vi "NIDCPower_channel_ganging - check channel list_full config.vi"(8 "error in (no error)":errorcluster, 11 "Channel List In":T1[](array[typedef])) -> (0 "error out":errorcluster, 3 "Channel List Out":T1[](array[typedef]))   [LabVIEW 2024]
uses:
  ctl/NIDCPower_channel_ganging - ctl - channel def.ctl
  ctl/NIDCPower_channel_ganging - ctl - channel mode.ctl
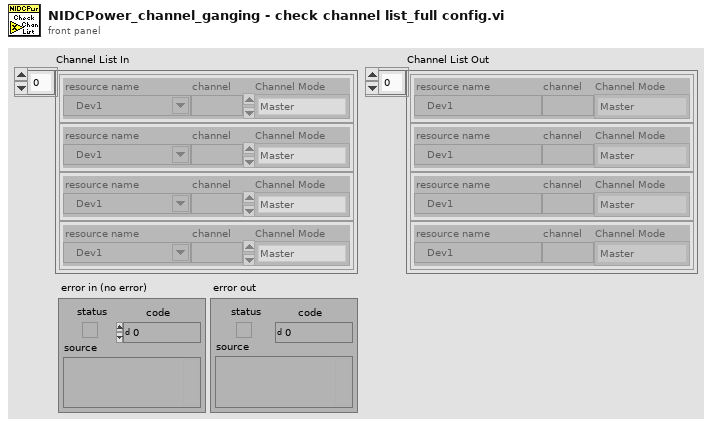
[diagram p1: front panel]
types:
  T1 = typedef "NIDCPower_channel_ganging - ctl - channel def.ctl" = cluster{"resource name":refnum<k15>, "channels":string, "Channel Mode":T2}
  T2 = typedef "NIDCPower_channel_ganging - ctl - channel mode.ctl" = enum32{"Master", "Slave", "Slave - Inverted"}
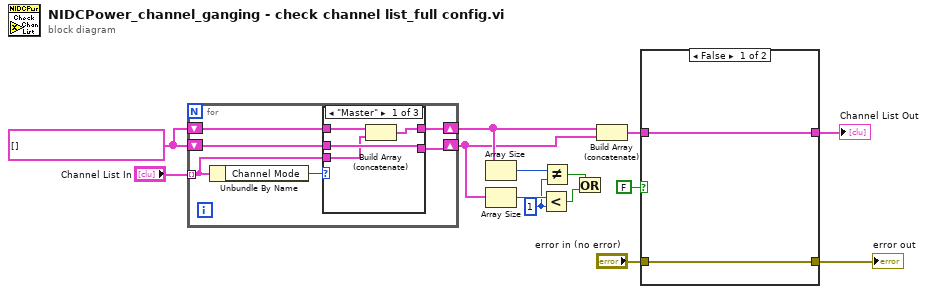
[diagram p0: block diagram]
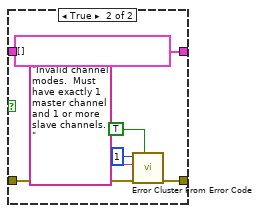
[diagram p2: hidden frame]
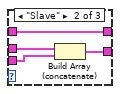
[diagram p3: hidden frame]
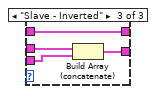
[diagram p4: hidden frame]
diagram:
  w10 = 1 ("y")
  w13 = T1[] [] ("Channel List")
  n1 = for {
    tunnel: "Channel List In" -> [w16] mode=indexing
    shift-right: [w15] -> w6
    shift-left: w13 -> [w17]
    shift-right: [w18] -> w7
    shift-left: w13 -> [w19]
    n2 = Unbundle By Name(w16) -> ("Channel Mode"=w20:T2)
    n3 = case shown="\"Master\"" w20 {
      tunnel: w19 -> [w23 w28 w32]
      tunnel: [w22 w28 w32] -> w18
      tunnel: w17 -> [w24 w27 w31]
      tunnel: w16 -> [w21 w26 w30]
      tunnel: [w24 w25 w29] -> w15
      frame "Master" {
        n4 = Build Array (concatenate)(w23, w21) -> (w22:T1[])
      }
      frame "Slave" {
        n5 = Build Array (concatenate)(w27, w26) -> (w25:T1[])
      }
      frame "Slave - Inverted" {
        n6 = Build Array (concatenate)(w31, w30) -> (w29:T1[])
      }
    }
  }
  n7 = Array Size(array=w7) -> (size(s)=w11:i32)
  n8 = Array Size(array=w6) -> (size(s)=w12:i32)
  n9 = Less?(x=w12, y=w10) -> (x < y?=w8:bool)
  n10 = Not Equal?(x=w11, y=w10) -> (x != y?=w9:bool)
  n11 = Or(x=w9, y=w8) -> ()  [unwired: 1 out]
  n12 = Build Array (concatenate)(w7, w6) -> (w5:T1[])
  n13 = case shown="False" FALSE {
    tunnel: w5 -> [w34 _]
    tunnel: [w33 w40] -> w4
    tunnel: "error in (no error)" -> [w33 w39]
    tunnel: [w34 T1[] []] -> w2
    frame False {
    }
    frame True {
      n14 = call <vilib>:"Error Cluster From Error Code.vi"("show call chain? (False)"=TRUE, "error in (no error)"=w39, "error message (\"\")"="Invalid channel modes.  Must have exactly 1 master channel and 1 or more slave channels." ("error message (\"\")"), "error code (0)"=1) -> ("error out"=w40:errorcluster)  [unwired: 5 in]
    }
  }
  "error out" <- w4
  "Channel List Out" <- w2
